vi "Lookup Base Protocol Class and Info.vi"(8 "error in (no error)":errorcluster, 10 "Protocol in":string, 11 "Class Lookup":variant) -> (0 "error out":errorcluster, 1 "Protocol out":T1, 2 "Protocol Parent out":refnum<class "Protocol Parent.lvclass">, 3 "Class Lookup out":variant, 4 "Error Codes":cluster{"Code":i32, "String":string}[](array[cluster]))   [LabVIEW 2020, in "Instrument Addon Shared.lvlib"]
uses:
  Instrument Addon Shared.lvlib
  Libraries Directory/Protocols.lvlibp/Protocol Parent/Protocol Parent.lvclass
  Libraries Directory/Protocols.lvlibp/Protocol Parent/Types/Base Protocol Type.ctl
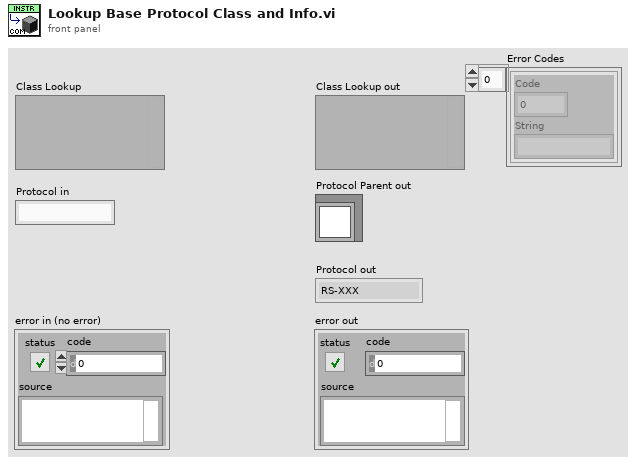
[diagram p1: front panel]
types:
  T1 = typedef "Protocols.lvlibp/Protocol Parent.lvclass/Base Protocol Type.ctl" = enum16{"RS-XXX", "VISA", "TCPIP", "UDP", "GPIB ConvBox"}
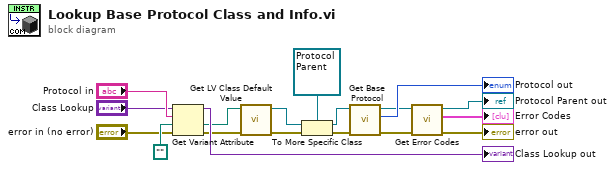
[diagram p0: block diagram]
diagram:
  n1 = Get Variant Attribute(Variant="Class Lookup", name="Protocol in", default value (empty Variant)=path "", error in="error in (no error)") -> (duplicate Variant=→"Class Lookup out":variant, value=w10:path, error out=w11:errorcluster)  [unwired: 1 out]
  n2 = call <vilib>:"Get LV Class Default Value.vi"("error in (no error)"=w11, "class path"=w10) -> ("error out"=w12:errorcluster, "object"=w15:refnum<class>)  [unwired: 8 in]
  n3 = To More Specific Class(target class=refnum<class "Protocol Parent.lvclass"> refnum ("Protocols.lvlibp:Protocol Parent.lvclass"), reference=w15, error in=w12) -> (specific class reference=w16:refnum<class "Protocol Parent.lvclass">, error out=w13:errorcluster)
  n4 = call-dynamic "Get Base Protocol.vi"("error in (no error)"=w13, "Protocol Parent in"=w16) -> ("error out"=w5:errorcluster, "Protocol out"=→"Protocol out":T1, "Protocol Parent out"=w4:refnum<class "Protocol Parent.lvclass">)  [unwired: 7 in]
  n5 = call-dynamic "Get Error Codes.vi"("error in (no error)"=w5, "Protocol Parent in"=w4) -> ("error out"=→"error out":errorcluster, "Error Codes"=→"Error Codes":cluster{"Code":i32, "String":string}[], "Protocol Parent out"=→"Protocol Parent out":refnum<class "Protocol Parent.lvclass">)  [unwired: 7 in]
